vi "User Interface.vi"(8 "error in":errorcluster, 10 "User Event References":T4) -> (0 "error out":errorcluster)   [LabVIEW 2015]
uses:
  TypeDef/User Event References.ctl
  TypeDef/GetData Cluster.ctl
  TypeDef/ResultUpdate Cluster.ctl
  TypeDef/Initialize_Cluster.ctl
  TypeDef/OverWrite JSON Cluster.ctl
  TypeDef/GraphReff.ctl
  <vilib>/event_ctls.llb/usereventprio.ctl
panel:
  in  "Cp-CpkTable":string[][](table)=[["1.13", "1.14", "1.13", "1.16", "1.18"], ["1.14", "1.12", "1.12", "1.01", "1.02"], ["1.29", "1.26", "1.26", "1.03", "1.04"], ["0.10", "0.10", "0.13", "0.13", "0.11"], ["-0.05", "-0.10", "-0.17", "-0.07", "-0.22"]]
  out "Histogram Summary 5":T1(graph) caption="Measurement5 Histogram summary"
  out "Histogram Summary 4":T1(graph) caption="Measurement4 Histogram summary"
  out "Histogram Summary 3":T1(graph) caption="Measurement3 Histogram summary"
  out "Histogram Summary 2":T1(graph) caption="Measurement2 Histogram summary"
  out "Bar graph 2":dbl[][](graph) caption="Defect Summary"
  out "defect":picture caption="Defect Chart"
  out "yeild":picture caption="Yeild Chart"
  out "Measurement-Summary -1 5":T2(graph)={"Start"=1, "index"=0, "Waveform Graph"=[]} caption="Measurement5 summary"
  out "Measurement-Summary -1 4":T2(graph)={"Start"=1, "index"=0, "Waveform Graph"=[]} caption="Measurement4 summary"
  out "Measurement-Summary -1 3":T2(graph)={"Start"=1, "index"=0, "Waveform Graph"=[]} caption="Measurement3 summary"
  out "Measurement-Summary -1 2":T2(graph)={"Start"=1, "index"=0, "Waveform Graph"=[]} caption="Measurement2 summary"
  out "Measurement-Summary -1":T2(graph)={"Start"=1, "index"=0, "Waveform Graph"=[]} caption="Measurement1 summary"
  out "Lable 2":picture
  out "Lable":picture caption="Lable 2"
  out "Bar graph":dbl[][](graph) caption="Production Summary"
  out "Histogram Summary":T1(graph) caption="Measurement1 Histogram summary"
  in  "Cluster Of Graphs":T3
  out "Defect":bool[](array[boolean])
  out "isPass":bool
  out "Result Upd":bool
  out "Terminal Count":u32
  out "Terminal Data 1D":dbl[](array[numeric])
  in  "BACK":bool
  in  "EXIT":bool
  in  "ANALYTICS":bool
  in  "STOP":bool
  in  "PAUSE":bool
  in  "RUN":bool
  # "ANALYTICS DASHBOARD"
  # "Result Update Test Bench"
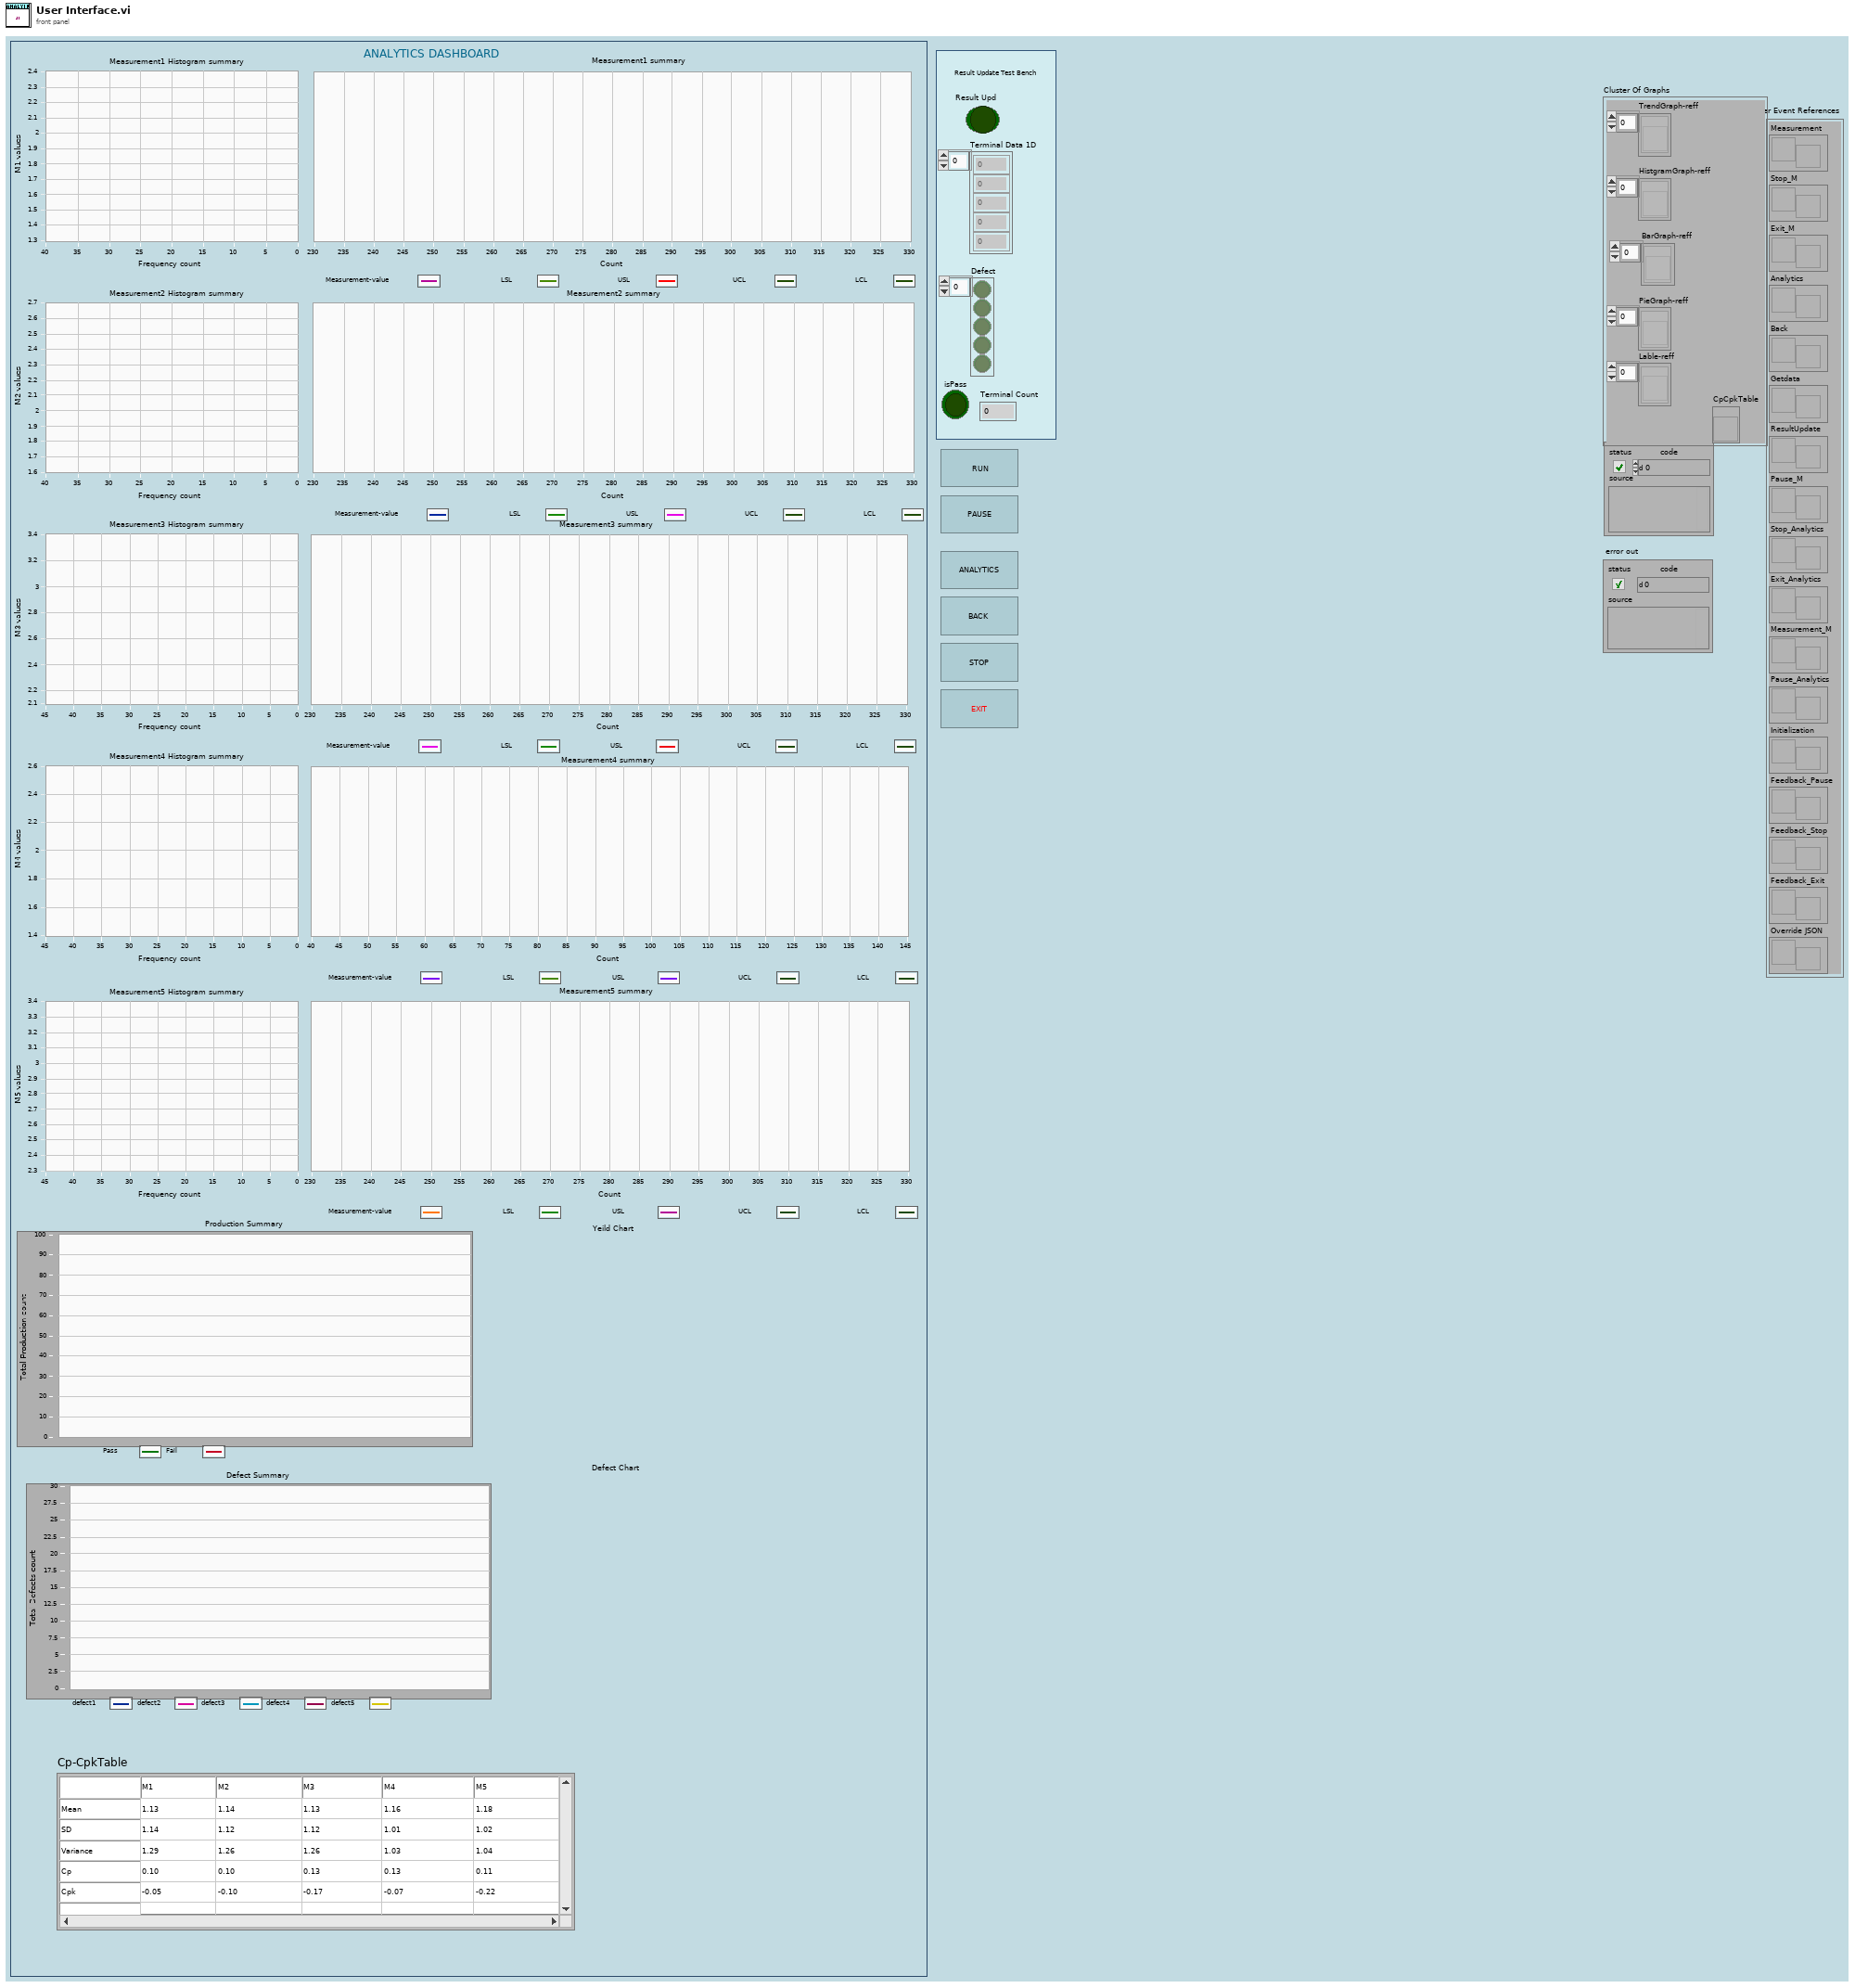
[diagram p1: front panel]
types:
  T1 = cluster{"X Values":dbl[], "Best Gaussian Fit":dbl[]}[]
  T2 = cluster{"Start":i32, "index":i32, "Waveform Graph":dbl[][]}
  T3 = typedef "GraphReff.ctl" = cluster{"HistgramGraph-reff":refnum<vi>[], "BarGraph-reff":refnum<vi>[], "PieGraph-reff":refnum<vi>[], "Lable-reff":refnum<vi>[], "TrendGraph-reff":refnum<vi>[], "CpCpkTable":refnum<vi>}
  T4 = typedef "User Event References.ctl" = cluster{"Measurement":refnum<user-event>, "Stop_M":refnum<user-event>, "Exit_M":refnum<user-event>, "Analytics":refnum<user-event>, "Back":refnum<user-event>, "Getdata":refnum<user-event>, "ResultUpdate":refnum<user-event>, "Pause_M":refnum<user-event>, "Stop_Analytics":refnum<user-event>, "Exit_Analytics ":refnum<user-event>, "Measurement_M":refnum<user-event>, "Pause_Analytics":refnum<user-event>, "Initialization":refnum<user-event>, "Feedback_Pause":refnum<user-event>, "Feedback_Stop":refnum<user-event>, "Feedback_Exit":refnum<user-event>, "Override JSON":refnum<user-event>}
  T5 = typedef "usereventprio.ctl" = enum32{"high priority", "normal priority"}
  T6 = typedef "OverWrite JSON Cluster.ctl" = cluster{"JSON Path":path}
  T7 = typedef "GetData Cluster.ctl" = cluster{"Terminal Count":u32, "isPass":bool, "Terminal Data 1D":dbl[], "Defect":bool[]}
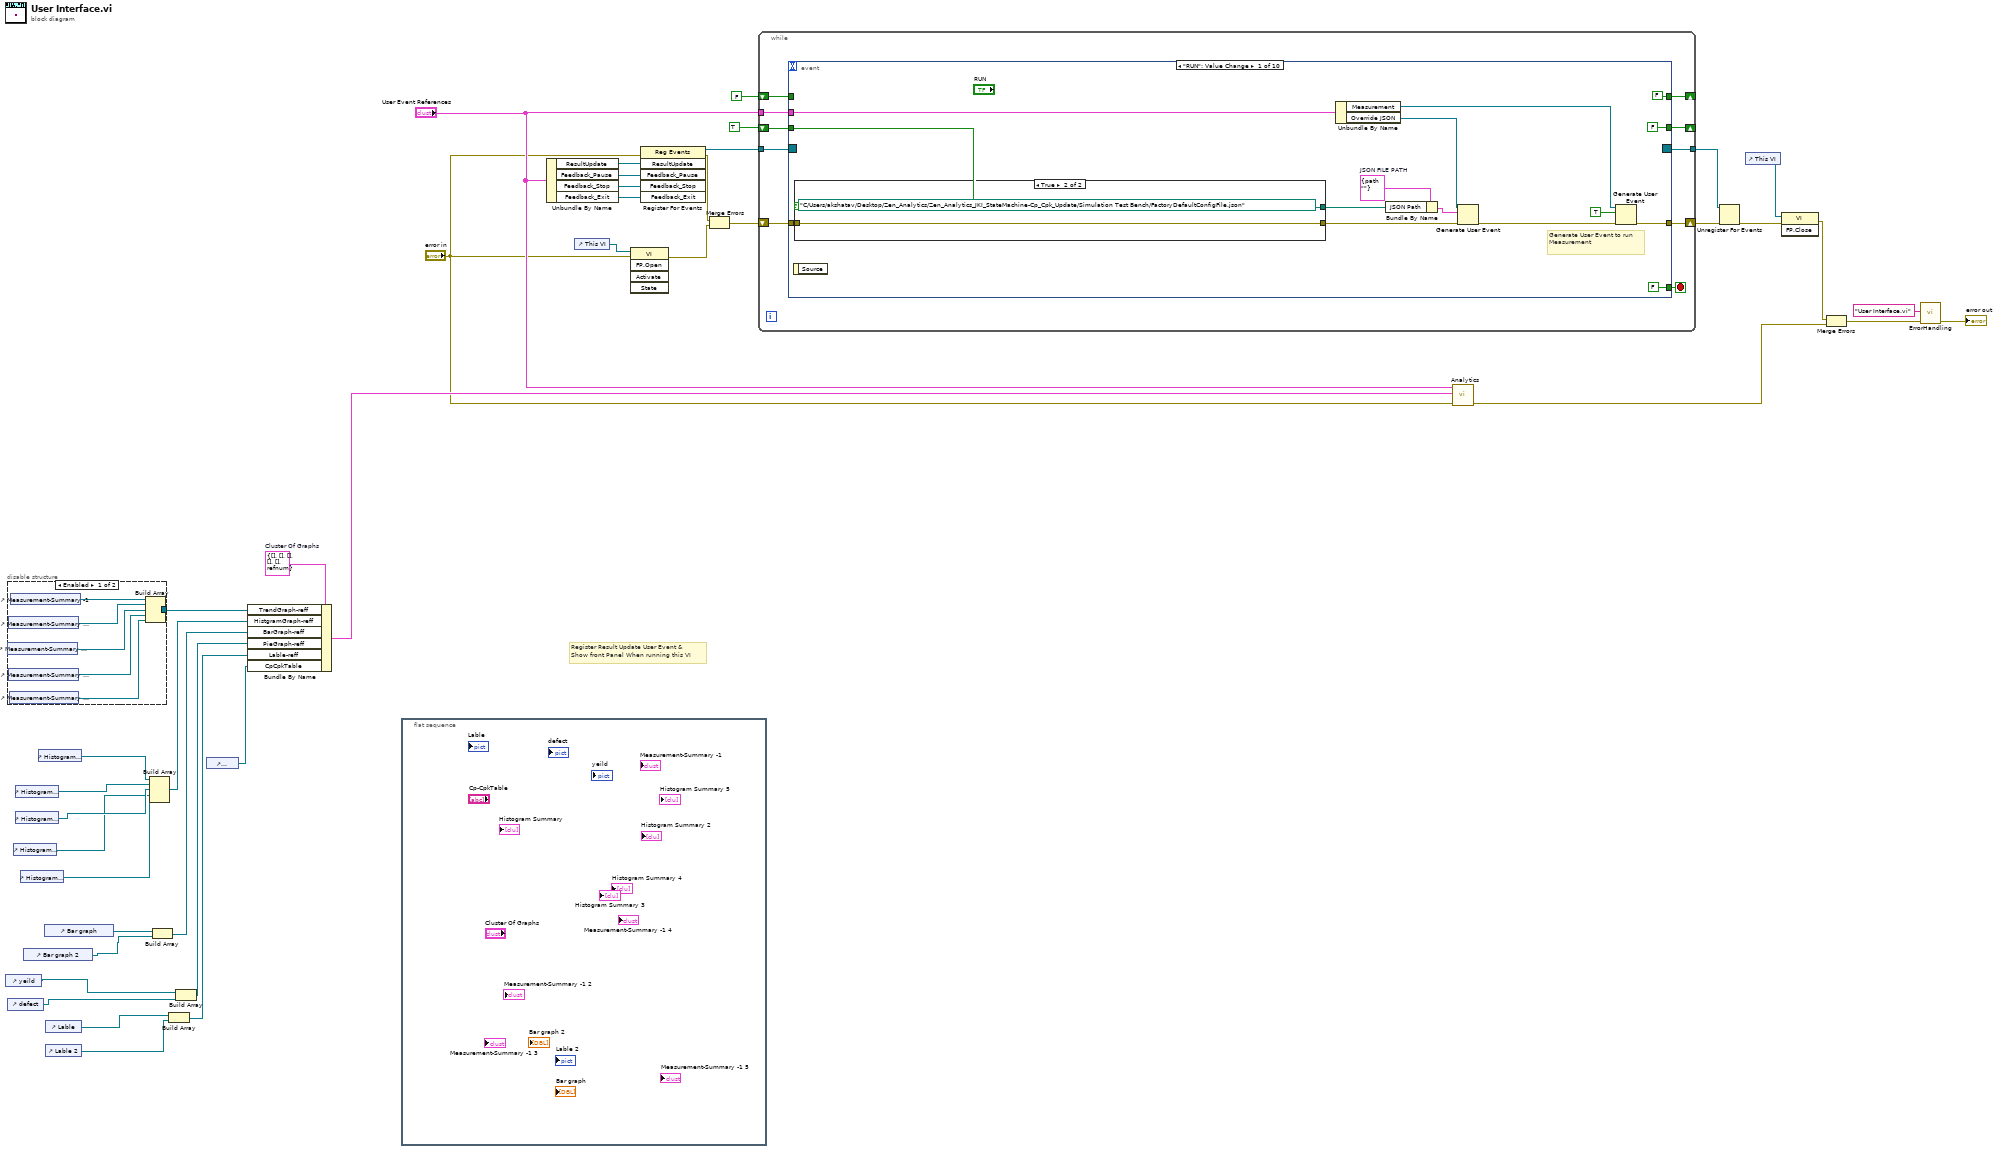
[diagram p0: block diagram]
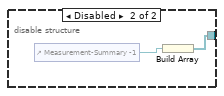
[diagram p2: hidden frame]
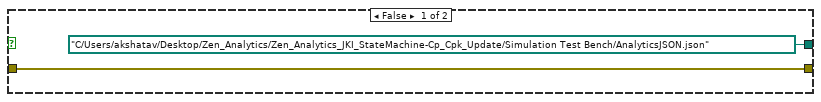
[diagram p3: hidden frame]
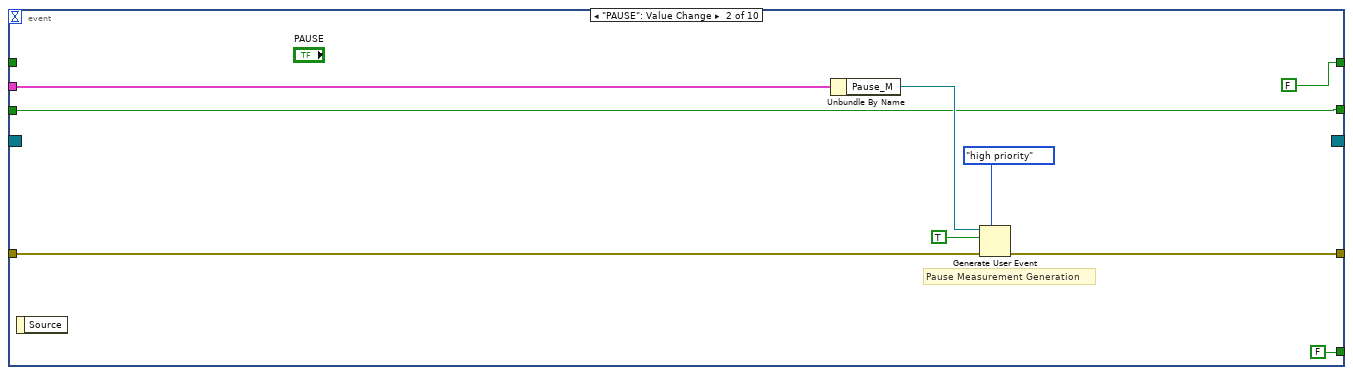
[diagram p4: hidden frame]
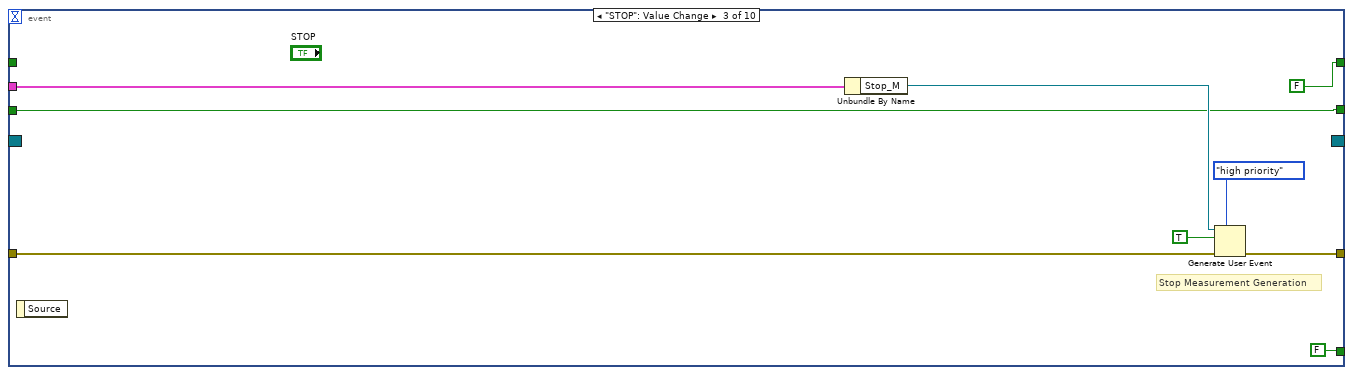
[diagram p5: hidden frame]
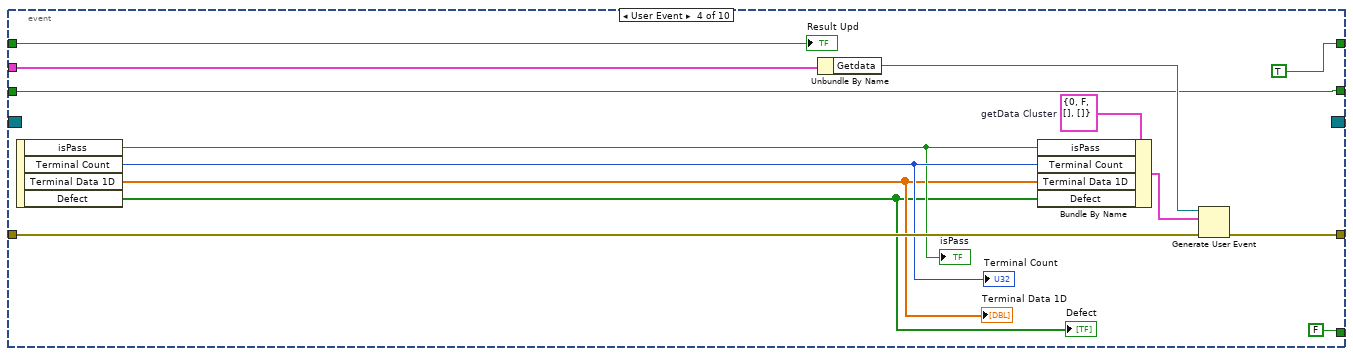
[diagram p6: hidden frame]
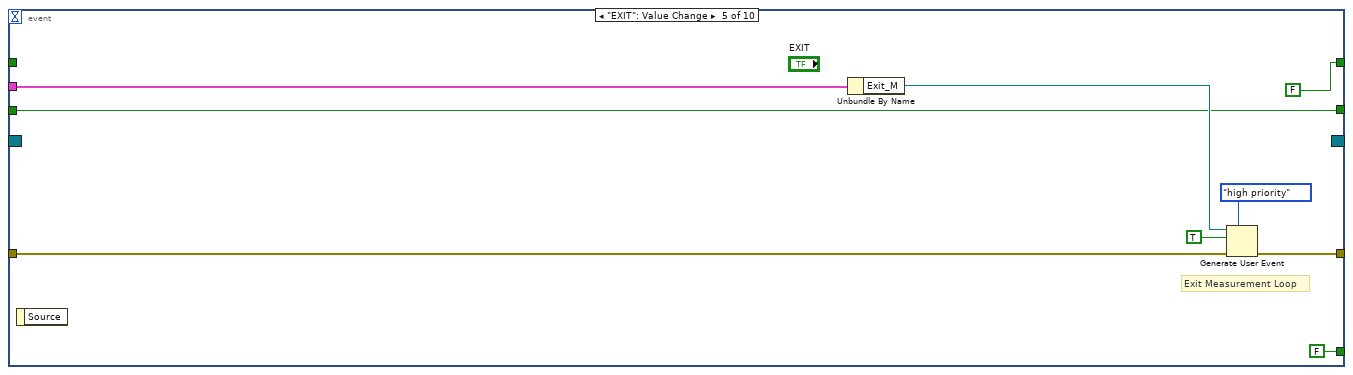
[diagram p7: hidden frame]
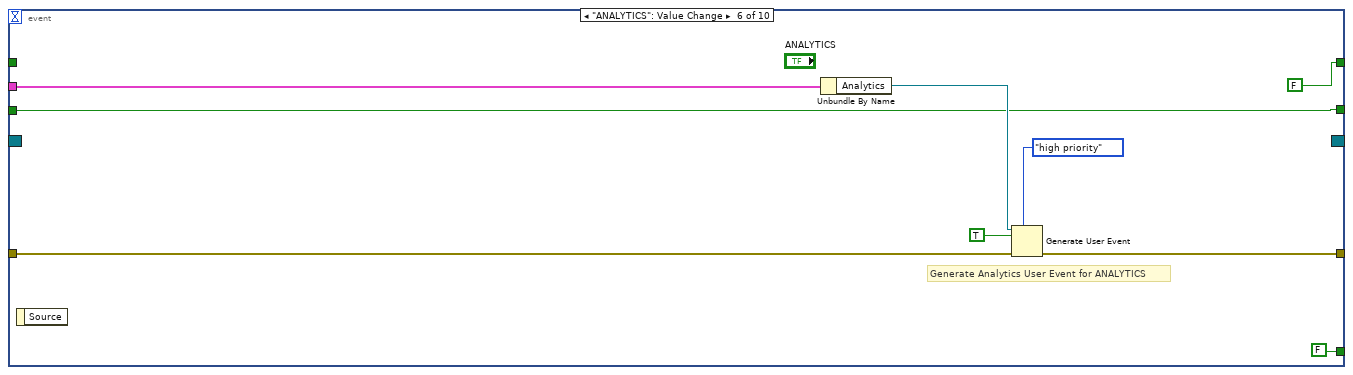
[diagram p8: hidden frame]
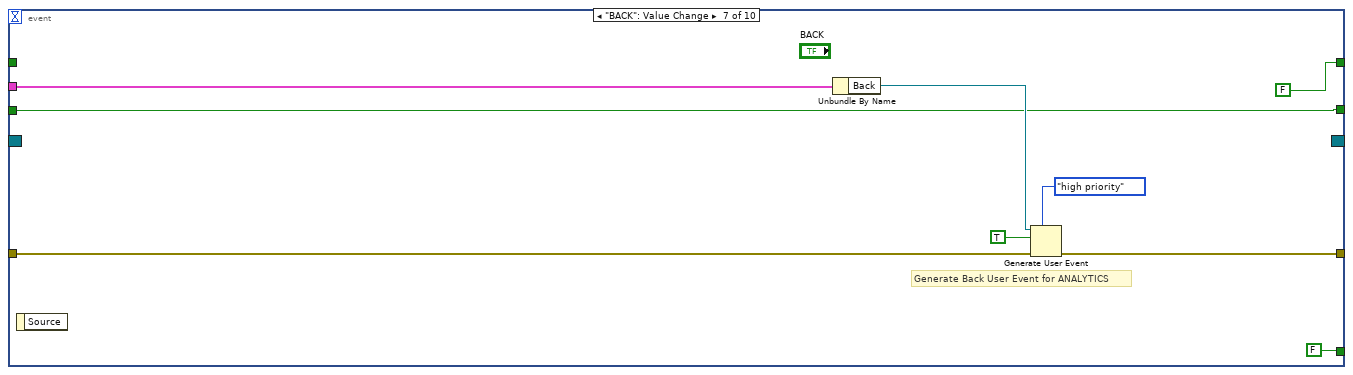
[diagram p9: hidden frame]
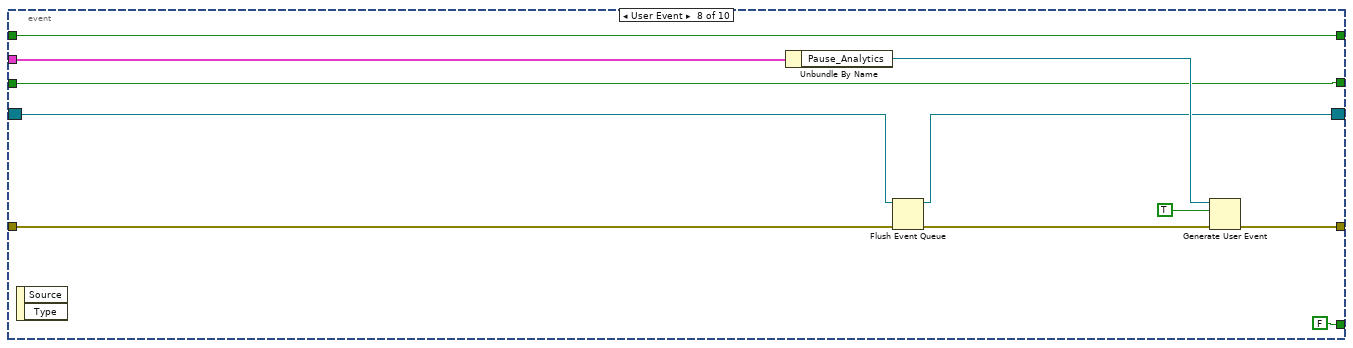
[diagram p10: hidden frame]
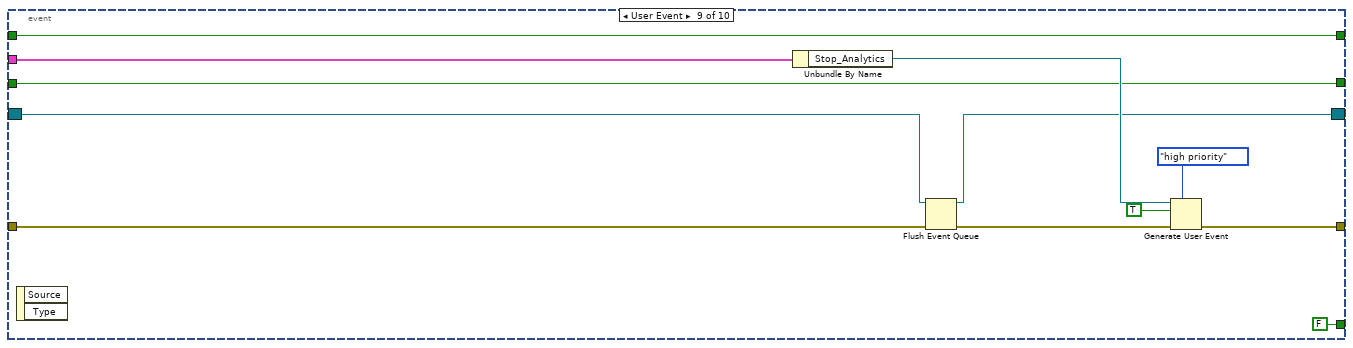
[diagram p11: hidden frame]
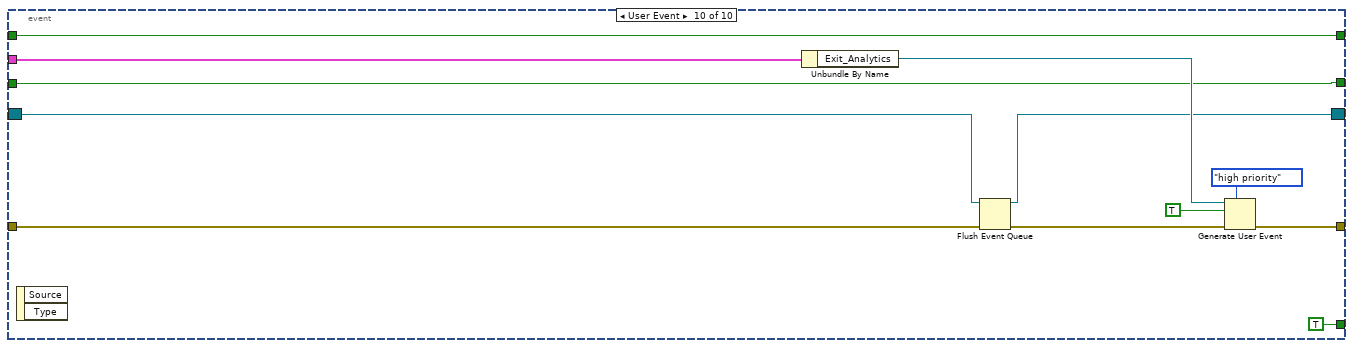
[diagram p12: hidden frame]
diagram:
  w24 = T3 {"HistgramGraph-reff"=[], "BarGraph-reff"=[], "PieGraph-reff"=[], "Lable-reff"=[], "TrendGraph-reff"=[], "CpCpkTable"=refnum}  # Cluster Of Graphs
  # "Register Result Update User Event &\nShow front Panel When running this VI"
  n1 = control-ref of="yeild"() -> (w10:refnum<vi>)
  n2 = disable-structure shown="Enabled" {
    disable-tunnel: [w46 w49] -> w11
    frame Enabled {
      n3 = control-ref of="Measurement-Summary -1 3"() -> (w44:refnum<vi>)
      n4 = control-ref of="Measurement-Summary -1 2"() -> (w45:refnum<vi>)
      n5 = control-ref of="Measurement-Summary -1 4"() -> (w43:refnum<vi>)
      n6 = control-ref of="Measurement-Summary -1 5"() -> (w42:refnum<vi>)
      n7 = control-ref of="Measurement-Summary -1"() -> (w47:refnum<vi>)
      n8 = Build Array(w47, w45, w44, w43, w42) -> (w46:refnum<vi>[])
    }
    frame Disabled {
      n9 = control-ref of="Measurement-Summary -1"() -> (w48:refnum<vi>)
      n10 = Build Array(w48) -> (w49:refnum<vi>[])
    }
  }
  n11 = control-ref of="defect"() -> (w9:refnum<vi>)
  n12 = control-ref of="Histogram Summary 4"() -> (w5:refnum<vi>)
  n13 = control-ref of="Histogram Summary 3"() -> (w6:refnum<vi>)
  n14 = control-ref of="Histogram Summary 2"() -> (w7:refnum<vi>)
  n15 = control-ref of="Histogram Summary 5"() -> (w4:refnum<vi>)
  n16 = control-ref of="Bar graph 2"() -> (w8:refnum<vi>)
  n17 = control-ref of="Histogram Summary"() -> (w19:refnum<vi>)
  n18 = control-ref of="Bar graph"() -> (w18:refnum<vi>)
  n19 = control-ref of="Lable"() -> (w17:refnum<vi>)
  n20 = control-ref of="Lable 2"() -> (w16:refnum<vi>)
  n21 = Build Array(w19, w7, w6, w5, w4) -> (w15:refnum<vi>[])
  n22 = Build Array(w18, w8) -> (w14:refnum<vi>[])
  n23 = Build Array(w17, w16) -> (w12:refnum<vi>[])
  n24 = Build Array(w10, w9) -> (w13:refnum<vi>[])
  n25 = control-ref of="Cp-CpkTable"() -> (w3:refnum<vi>)
  n26 = Bundle By Name(cluster=w24, "TrendGraph-reff"=w11, "HistgramGraph-reff"=w15, "BarGraph-reff"=w14, "PieGraph-reff"=w13, "Lable-reff"=w12, "CpCpkTable"=w3) -> (w23:T3)
  n27 = flat-sequence {
    frame #0 {
    }
  }
  n28 = Unbundle By Name("User Event References") -> ("ResultUpdate"=w40:refnum<user-event>, "Feedback_Pause"=w27:refnum<user-event>, "Feedback_Stop"=w26:refnum<user-event>, "Feedback_Exit"=w25:refnum<user-event>)
  n29 = control-ref of="This VI"() -> (w37:refnum<vi>)
  n30 = invoke class="VI" method="FP.Open"(reference=w37, error in="error in") -> (error out=w35:errorcluster)  [unwired: 3 in, 4 out]
  n31 = register-events(error in="error in", w40, w27, w26, w25) -> (reference out=w41:refnum<event-registration>, error out=w36:errorcluster)  [unwired: 1 in]
  n32 = Merge Errors(w36, w35) -> (w34:errorcluster)
  n33 = while {
    shift-right: [w58] -> w30
    shift-left: w34 -> [w59]
    tunnel: "User Event References" -> [w57]
    tunnel: w41 -> [w55]
    shift-right: [w54] -> _
    shift-left: FALSE -> [w52]
    tunnel: [w53] -> w28
    shift-right: [w51] -> _
    shift-left: TRUE -> [w50]
    stop <- w56 stop-if-true
    n34 = event shown="[0] \"RUN\": Value Change" {
      selector: w55 -> [_ _ _ _ _ _ _ w143 w156 w164]
      dyn-events: [_ _ _ _ _ _ _ w142 w155 w163] -> w53
      timeout: _ -> [_ _ _ _ _ _ _ _ _ _]
      tunnel: w59 -> [w65 w86 w89 w108 w112 w128 w137 w141 w154 w166]
      tunnel: [w70 w80 w90 w107 w113 w127 w136 w139 w152 w165] -> w58
      tunnel: w57 -> [w74 w87 w96 w106 w118 w126 w135 w146 w159 w167]
      tunnel: [FALSE FALSE FALSE FALSE FALSE FALSE FALSE FALSE FALSE TRUE] -> w56
      tunnel: [FALSE FALSE FALSE TRUE FALSE FALSE FALSE w147 w150 w162] -> w54
      tunnel: w52 -> [_ _ _ w98 _ _ _ w147 w150 w162]
      tunnel: [FALSE w79 w88 w97 w111 w120 w129 w138 w149 w161] -> w51
      tunnel: w50 -> [w66 w79 w88 w97 w111 w120 w129 w138 w149 w161]
      event "RUN": Value Change {
        w63 = T6 {"JSON Path"=path ""}  # JSON FILE PATH
        # "Generate User Event to run Measurement"
        n35 = event-data() -> ()  [unwired: 1 in, 1 out]
        n36 = case shown="True" w66 {
          tunnel: [path "C:/Users/akshatav/Desktop/Zen_Analytics/Zen_Analytics_JKI_StateMachine-Cp_Cpk_Update/Simulation Test Bench/AnalyticsJSON.json" ("file (use dialog)") path "C:/Users/akshatav/Desktop/Zen_Analytics/Zen_Analytics_JKI_StateMachine-Cp_Cpk_Update/Simulation Test Bench/FactoryDefaultConfigFile.json" ("file (use dialog)")] -> w61
          tunnel: w65 -> [w75 w77]
          tunnel: [w75 w77] -> w62
          frame False {
          }
          frame True {
          }
        }
        n37 = Unbundle By Name(w74) -> ("Measurement"=w73:refnum<user-event>, "Override JSON"=w64:refnum<user-event>)
        n38 = Bundle By Name(cluster=w63, "JSON Path"=w61) -> (w60:T6)
        n39 = Generate User Event(user event=w64, event data cluster=w60, error in=w62) -> (error out=w68:errorcluster)  [unwired: 1 in, 1 out]
        n40 = Generate User Event(user event=w73, event data cluster=TRUE, error in=w68) -> (error out=w70:errorcluster)  [unwired: 1 in, 1 out]
      }
      event "PAUSE": Value Change {
        # "Pause Measurement Generation"
        n41 = event-data() -> ()  [unwired: 1 in, 1 out]
        n42 = Unbundle By Name(w87) -> ("Pause_M"=w84:refnum<user-event>)
        n43 = Generate User Event(priority (normal)=usereventprio."high priority", user event=w84, event data cluster=TRUE, error in=w86) -> (error out=w80:errorcluster)  [unwired: 1 out]
      }
      event "STOP": Value Change {
        # "Stop Measurement Generation"
        n44 = event-data() -> ()  [unwired: 1 in, 1 out]
        n45 = Unbundle By Name(w96) -> ("Stop_M"=w95:refnum<user-event>)
        n46 = Generate User Event(priority (normal)=usereventprio."high priority", user event=w95, event data cluster=TRUE, error in=w89) -> (error out=w90:errorcluster)  [unwired: 1 out]
      }
      event User Event {
        w104 = T7 {"Terminal Count"=0, "isPass"=FALSE, "Terminal Data 1D"=[], "Defect"=[]}  # getData Cluster
        n47 = event-data() -> ("isPass"=w101:bool, "Terminal Count"=w102:u32, "Terminal Data 1D"=w100:dbl[], "Defect"=w99:bool[])  [unwired: 1 in]
        "Terminal Count" <- w102
        "isPass" <- w101
        "Terminal Data 1D" <- w100
        "Defect" <- w99
        n48 = Unbundle By Name(w106) -> ("Getdata"=w105:refnum<user-event>)
        n49 = Bundle By Name(cluster=w104, "isPass"=w101, "Terminal Count"=w102, "Terminal Data 1D"=w100, "Defect"=w99) -> (w103:T7)
        n50 = Generate User Event(user event=w105, event data cluster=w103, error in=w108) -> (error out=w107:errorcluster)  [unwired: 1 in, 1 out]
        "Result Upd" <- w98
      }
      event "EXIT": Value Change {
        # "Exit Measurement Loop"
        n51 = event-data() -> ()  [unwired: 1 in, 1 out]
        n52 = Unbundle By Name(w118) -> ("Exit_M"=w117:refnum<user-event>)
        n53 = Generate User Event(priority (normal)=usereventprio."high priority", user event=w117, event data cluster=TRUE, error in=w112) -> (error out=w113:errorcluster)  [unwired: 1 out]
      }
      event "ANALYTICS": Value Change {
        # "Generate Analytics User Event for ANALYTICS"
        n54 = event-data() -> ()  [unwired: 1 in, 1 out]
        n55 = Unbundle By Name(w126) -> ("Analytics"=w125:refnum<user-event>)
        n56 = Generate User Event(priority (normal)=usereventprio."high priority", user event=w125, event data cluster=TRUE, error in=w128) -> (error out=w127:errorcluster)  [unwired: 1 out]
      }
      event "BACK": Value Change {
        # "Generate Back User Event for ANALYTICS"
        n57 = event-data() -> ()  [unwired: 1 in, 1 out]
        n58 = Unbundle By Name(w135) -> ("Back"=w134:refnum<user-event>)
        n59 = Generate User Event(priority (normal)=usereventprio."high priority", user event=w134, event data cluster=TRUE, error in=w137) -> (error out=w136:errorcluster)  [unwired: 1 out]
      }
      event User Event {
        n60 = event-data() -> ()  [unwired: 1 in, 2 out]
        n61 = Unbundle By Name(w146) -> ("Pause_Analytics"=w145:refnum<user-event>)
        n62 = Flush Event Queue(0:w143, 3:w141) -> (8:w142:refnum<event-registration>, 11:w140:errorcluster)  [unwired: 4 in, 1 out]
        n63 = Generate User Event(user event=w145, event data cluster=TRUE ("event data"), error in=w140) -> (error out=w139:errorcluster)  [unwired: 1 in, 1 out]
      }
      event User Event {
        n64 = event-data() -> ()  [unwired: 1 in, 2 out]
        n65 = Unbundle By Name(w159) -> ("Stop_Analytics"=w158:refnum<user-event>)
        n66 = Flush Event Queue(0:w156, 3:w154) -> (8:w155:refnum<event-registration>, 11:w153:errorcluster)  [unwired: 4 in, 1 out]
        n67 = Generate User Event(priority (normal)=usereventprio."high priority", user event=w158, event data cluster=TRUE ("event data"), error in=w153) -> (error out=w152:errorcluster)  [unwired: 1 out]
      }
      event User Event {
        n68 = event-data() -> ()  [unwired: 1 in, 2 out]
        n69 = Unbundle By Name(w167) -> ("Exit_Analytics"=w171:refnum<user-event>)
        n70 = Flush Event Queue(0:w164, 3:w166) -> (8:w163:refnum<event-registration>, 11:w169:errorcluster)  [unwired: 4 in, 1 out]
        n71 = Generate User Event(priority (normal)=usereventprio."high priority", user event=w171, event data cluster=TRUE ("event data"), error in=w169) -> (error out=w165:errorcluster)  [unwired: 1 out]
      }
    }
  }
  n72 = call "Analytics.vi"("error in"="error in", "Cluster Of Graphs"=w23, "User Event References"="User Event References") -> ("error out"=w1:errorcluster)  [unwired: 8 in]
  n73 = Unregister For Events(event registration refnum=w28, error in=w30) -> (error out=w29:errorcluster)
  n74 = control-ref of="This VI"() -> (w33:refnum<vi>)
  n75 = invoke class="VI" method="FP.Close"(reference=w33, error in=w29) -> (error out=w32:errorcluster)  [unwired: 1 in, 2 out]
  n76 = Merge Errors(w32, w1) -> (w38:errorcluster)
  n77 = call "ErrorHandling.vi"("error in (no error)"=w38, "Vi-name"="User Interface.vi") -> ("error out"=→"error out":errorcluster)  [unwired: 9 in]
